vi "TDT-Initialize Down Ramp.vi"(0 "RPcoX in":refnum<k7>, 7 "Ramp (ms)":dbl=20.0, 9 "Fs (Hz)":dbl, 11 "error in (no error)":errorcluster) -> (4 "RPcoX out":refnum<k7>, 15 "error out":errorcluster)   [LabVIEW 2020]
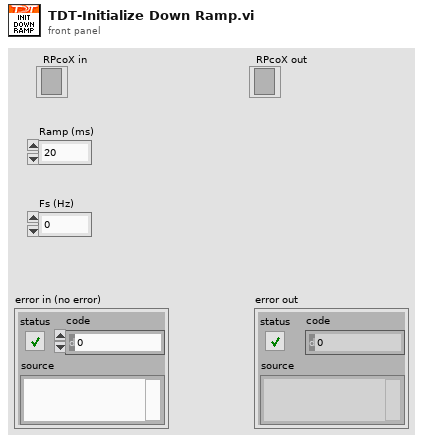
[diagram p1: front panel]
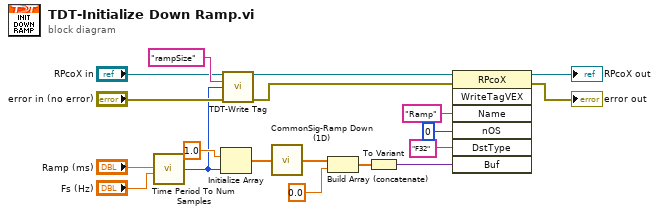
[diagram p0: block diagram]
diagram:
  n1 = call "Time Period To Num Samples.vi"("Duration (ms)"="Ramp (ms)", "Sampling rate (Hz)"="Fs (Hz)") -> ("Samples"=w3:i32)  [unwired: 5 in]
  n2 = Initialize Array(1.0, w3) -> (w9:dbl[])
  n3 = call "TDT-Write Tag.vi"("RPcox"="RPcoX in", "Name"="rampSize", "Value"=w3, "error in"="error in (no error)") -> ("RPcox Out"=w13:refnum<k7>, "error out"=w16:errorcluster)  [unwired: 10 in]
  n4 = call "CommonSig-Ramp Down (1D).vi"("Array"=w9) -> ("Ramped array"=w7:dbl[])  [unwired: 4 in]
  n5 = Build Array (concatenate)(w7, 0.0) -> (w2:dbl[])
  n6 = To Variant(anything=w2) -> (Variant=w6:variant)
  n7 = invoke class="RPcoX" method="WriteTagVEX"(reference=w13, error in=w16, "Name"="Ramp", "nOS"=0, "DstType"="F32", "Buf"=w6) -> (reference out=→"RPcoX out":refnum<k7>, error out=→"error out":errorcluster)  [unwired: 1 in, 5 out]
